vi "mainUIPumpProbe.vi"() -> ()   [LabVIEW 2017]
uses:
  globalUtilities.vi
  globalDevices.vi
panel:
  in  "axis (z)":u16(ring)=2 items=["x", "y", "z"]
  in  "length 2":i32
  in  "index 2":i32
  in  "length":i32
  in  "index":i32
  out "Waveform Graph":dbl[](graph)
  in  "saveVolume":bool
  in  "axis 1":u16(ring) items=["x", "y", "z"]
  out "frame 3":u64[][](graph)
  out "dropped frames":i32
  in  "acquisitionStart":bool
  in  "STOP":bool
  out "frame":u64[][](graph)
  in  "volume height (um)":dbl=80.0
  in  "volumes per second":dbl=0.5
  in  "GUI update divider":i32=1
  in  "frames per second":dbl=10.0
  out "folder name":string
  # "This VI sets all the acquisition parameters, starts the actual backend VI asynchronously, and displays the frames."
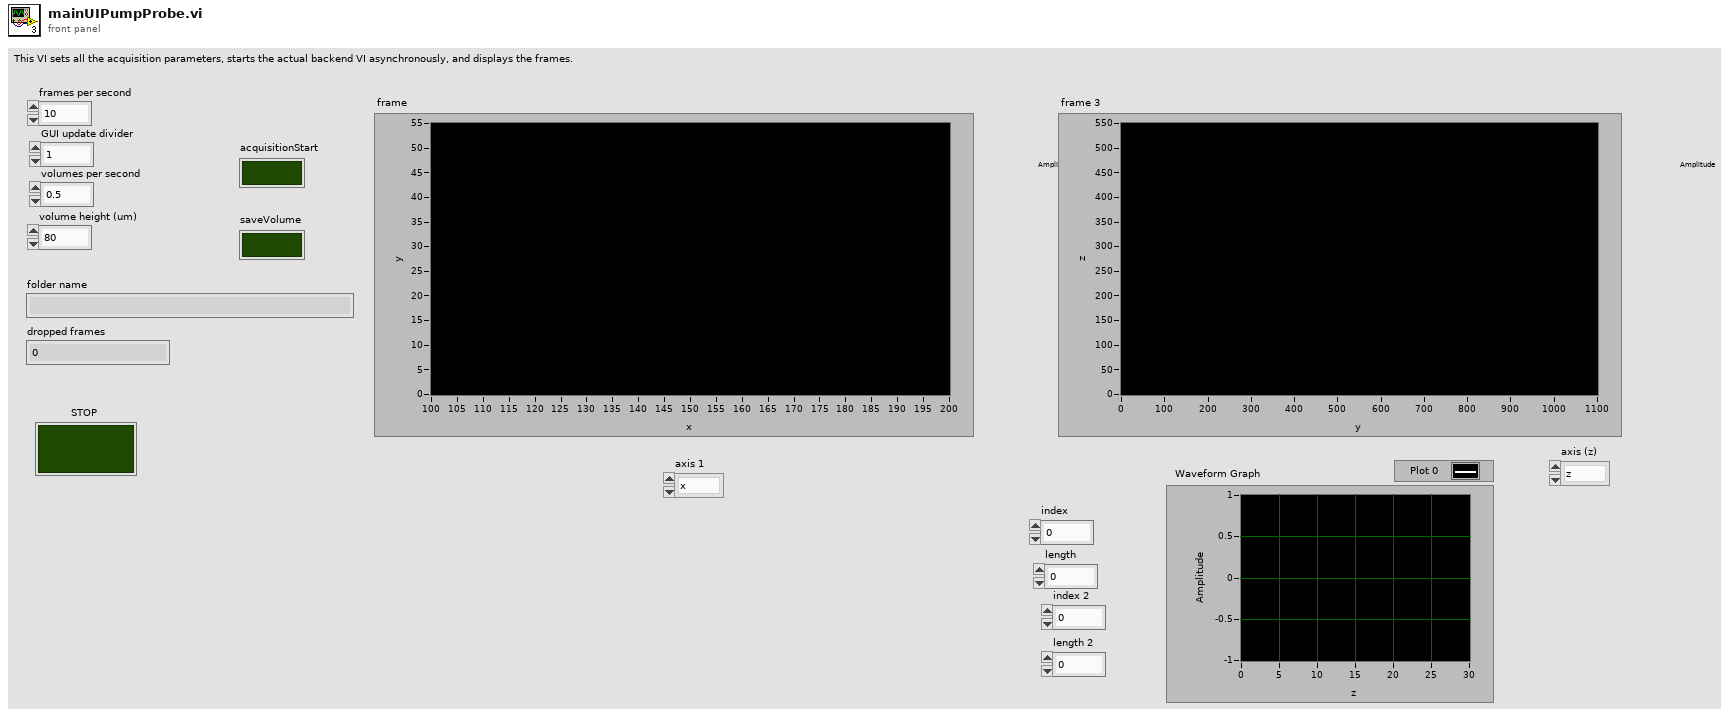
[diagram p1: front panel]
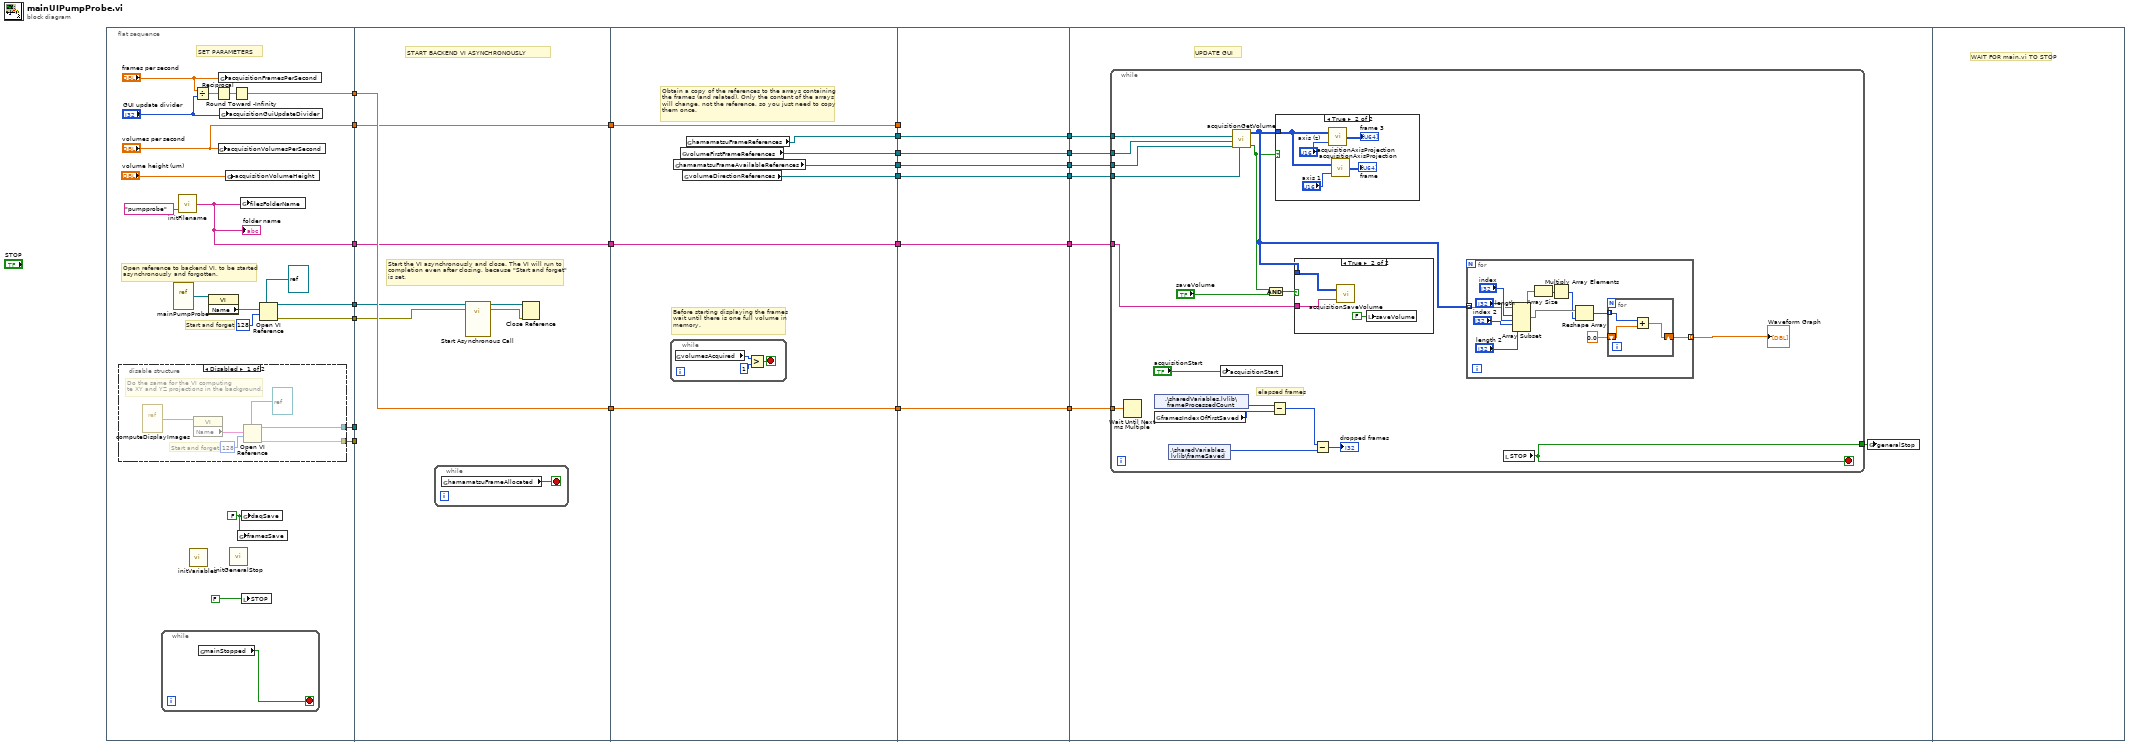
[diagram p0: block diagram]
diagram:
  n1 = flat-sequence {
    tunnel: [w37] -> w23
    tunnel: [w35] -> w22
    tunnel: [w33] -> w21
    tunnel: ["volumes per second"] -> w19
    tunnel: [w30] -> w17
    tunnel: [w29] -> w16
    tunnel: [w28] -> w15
    tunnel: w23 -> [w56]
    tunnel: [w56] -> w14
    tunnel: w22 -> [w55]
    tunnel: w21 -> [w54]
    tunnel: [w51] -> w12
    tunnel: w19 -> [w51]
    tunnel: [w50] -> w10
    tunnel: w17 -> [w50]
    tunnel: w16 -> [_]
    tunnel: w15 -> [_]
    tunnel: w14 -> [w64]
    tunnel: [w64] -> w13
    tunnel: w12 -> [w63]
    tunnel: [w63] -> w11
    tunnel: w10 -> [w62]
    tunnel: [w62] -> w9
    tunnel: [w61] -> w7
    tunnel: [w60] -> w5
    tunnel: [w59] -> w3
    tunnel: [w58] -> w1
    tunnel: w13 -> [w73]
    tunnel: [w73] -> w20
    tunnel: w11 -> [_]
    tunnel: [w72] -> w18
    tunnel: w9 -> [w72]
    tunnel: [w71] -> w8
    tunnel: w7 -> [w71]
    tunnel: [w70] -> w6
    tunnel: w5 -> [w70]
    tunnel: [w69] -> w4
    tunnel: w3 -> [w69]
    tunnel: [w68] -> w2
    tunnel: w1 -> [w68]
    tunnel: w20 -> [w80]
    tunnel: w18 -> [w78]
    tunnel: w8 -> [w77]
    tunnel: w6 -> [w76]
    tunnel: w4 -> [w75]
    tunnel: w2 -> [w74]
    frame #0 {
      w34 = FALSE ("daqSave")
      # "Start and forget"
      # "Open reference to backend VI, to be started\nasynchronously and forgotten."
      # "SET PARAMETERS"
      n2 = disable-structure shown="Disabled" {
        disable-tunnel: [w48 _] -> w29
        disable-tunnel: [w47 _] -> w28
        frame Disabled {
          # "Do the same for the VI computing\nte XY and YZ projections in the background."
          # "Start and forget"
          n3 = vi-ref "computeDisplayImages.vi"() -> (w43:refnum<vi>)
          n4 = property class="VI"(reference=w43) -> ("Name"=w46:string)  [unwired: 1 in, 2 out]
          n5 = Open VI Reference(type specifier VI Refnum (for type only)=refnum<vi> refnum, vi path=w46, options=128) -> (vi reference=w48:refnum<vi>, error out=w47:errorcluster)  [unwired: 3 in]
        }
        frame Enabled {
        }
      }
      n6 = while {
        stop <- w49 stop-if-true
        n7 = global read "globalUtilities.vi" "mainStopped"() -> (w49:bool)
      }
      n8 = vi-ref "mainPumpProbe.vi"() -> (w27:refnum<vi>)
      n9 = call "initFilename.vi"("Experiment type"="pumpprobe") -> ("folder name"=w30:string)  [unwired: 1 in]
      "folder name" <- w30
      n10 = call "initVariables.vi"() -> ()  [unwired: 12 in]
      n11 = Divide(x="frames per second", y="GUI update divider") -> (x/y=w39:dbl)
      n12 = property class="VI"(reference=w27) -> ("Name"=w26:string)  [unwired: 1 in, 2 out]
      n13 = Reciprocal(x=w39) -> (1/x=w38:dbl)
      n14 = global write "globalUtilities.vi" "acquisitionVolumesPerSecond"("volumes per second") -> ()
      n15 = global write "globalUtilities.vi" "acquisitionFramesPerSecond"("frames per second") -> ()
      n16 = global write "globalUtilities.vi" "acquisitionGuiUpdateDivider"("GUI update divider") -> ()
      n17 = global write "globalUtilities.vi" "acquisitionVolumeHeight"("volume height (um)") -> ()
      n18 = call "initGeneralStop.vi"() -> ()  [unwired: 1 in]
      n19 = Round Toward -Infinity(1:w38) -> (0:w37:dbl)
      n20 = global write "globalUtilities.vi" "framesSave"(w34) -> ()
      n21 = global write "globalUtilities.vi" "filesFolderName"(w30) -> ()
      n22 = local write "STOP"(FALSE) -> ()
      n23 = global write "globalUtilities.vi" "daqSave"(w34) -> ()
      n24 = Open VI Reference(type specifier VI Refnum (for type only)=refnum<vi> refnum, vi path=w26, options=128) -> (vi reference=w35:refnum<vi>, error out=w33:errorcluster)  [unwired: 3 in]
    }
    frame #1 {
      # "Start the VI asynchronously and close. The VI will run to\ncompletion even after closing, because \"Start and forget\"\nis set."
      # "START BACKEND VI ASYNCHRONOUSLY"
      n25 = while {
        stop <- w57 stop-if-true
        n26 = global read "globalDevices.vi" "hamamatsuFrameAllocated"() -> (w57:bool)
      }
      n27 = call-by-ref "Start Asynchronous Call"(reference=w55, error in=w54) -> (reference out=w53:refnum<vi>, error out=w52:errorcluster)  [unwired: 12 in]
      n28 = Close Reference(reference=w53, error in (no error)=w52) -> ()  [unwired: 1 out]
    }
    frame #2 {
      # "Obtain a copy of the references to the arrays containing \nthe frames (and related). Only the content of the arrays\nwill change, not the reference, so you just need to copy\nthem once."
      # "Before starting displaying the frames\nwait until there is one full volume in\nmemory."
      n29 = while {
        stop <- w66 stop-if-true
        n30 = global read "globalUtilities.vi" "volumesAcquired"() -> (w65:i32)
        n31 = Greater?(x=w65, y=1) -> (0:w66:bool)
      }
      n32 = global read "globalDevices.vi" "hamamatsuFrameAvailableReferences"() -> (w59:refnum<data-value>[])
      n33 = global read "globalUtilities.vi" "volumeFirstFrameReferences"() -> (w60:refnum<data-value>[])
      n34 = global read "globalUtilities.vi" "volumeDirectionReferences"() -> (w58:refnum<data-value>[])
      n35 = global read "globalDevices.vi" "hamamatsuFrameReferences"() -> (w61:refnum<data-value>[])
    }
    frame #3 {
    }
    frame #4 {
      # "UPDATE GUI"
      n36 = while {
        tunnel: w80 -> [w98]
        tunnel: [w91] -> w79
        tunnel: w78 -> [w90]
        tunnel: w77 -> [w87]
        tunnel: w76 -> [w86]
        tunnel: w75 -> [w85]
        tunnel: w74 -> [w84]
        stop <- w91 stop-if-true
        # "elapsed frames"
        n37 = Wait Until Next ms Multiple(millisecond multiple=w98) -> ()  [unwired: 1 out]
        n38 = shared-variable ".\\sharedVariables.lvlib\\frameProcessedCount"() -> (w96:i32)  [unwired: 1 in, 1 out]
        n39 = global read "globalUtilities.vi" "framesIndexOfFirstSaved"() -> (w95:i32)
        n40 = shared-variable ".\\sharedVariables.lvlib\\frameSaved"() -> (w93:u32)  [unwired: 1 in, 1 out]
        n41 = global write "globalUtilities.vi" "acquisitionStart"("acquisitionStart") -> ()
        n42 = call "acquisitionGetVolume.vi"("volumeDirectionReferences"=w84, "hamamatsuFrameAvailableReferences"=w85, "volumeFirstFrameReferences"=w86, "hamamatsuFrameReferences"=w87) -> ("success"=w81:bool, "volume out"=w89:u16[][][])  [unwired: 1 in, 3 out]
        n43 = And(x=w81, y="saveVolume") -> (x .and. y?=w83:bool)
        n44 = Subtract(x=w96, y=w95) -> (x-y=w94:i32)
        n45 = case shown="True" w81 {
          tunnel: w89 -> [_ w100]
          frame False {
          }
          frame True {
            n46 = call "acquisitionAxisProjection.vi"("axis (z)"="axis (z)", "z stack"=w100) -> ("projected img"=→"frame 3":u64[][])
            n47 = call "acquisitionAxisProjection.vi"("axis (z)"="axis 1", "z stack"=w100) -> ("projected img"=→"frame":u64[][])
          }
        }
        n48 = case shown="True" w83 {
          tunnel: w89 -> [_ w120]
          tunnel: w90 -> [_ w119]
          frame False {
          }
          frame True {
            n49 = call "acquisitionSaveVolume.vi"("folder"=w119, "volume"=w120) -> ()  [unwired: 1 in]
            n50 = local write "saveVolume"(FALSE ("saveVolume")) -> ()
          }
        }
        n51 = Subtract(x=w94, y=w93) -> (x-y=→"dropped frames":u32)
        n52 = for {
          tunnel: w89 -> [w110] mode=indexing
          tunnel: [w104] -> w88 mode=indexing
          n53 = Array Subset(array=w110, index (row)="index", length (row)="length", index (col)="index 2", length (col)="length 2") -> (w108:u16[][])
          n54 = Array Size(array=w108) -> (size(s)=w109:i32[])
          n55 = Multiply Array Elements(1:w109) -> (0:w107:i32)
          n56 = Reshape Array(w108, w107) -> (w106:u16[])
          n57 = for {
            tunnel: w106 -> [w117] mode=indexing
            shift-right: [w115] -> w104
            shift-left: 0.0 -> [w116]
            n58 = Add(x=w117, y=w116) -> (x+y=w115:dbl)
          }
        }
        "Waveform Graph" <- w88
        n59 = local read "STOP"() -> (w91:bool)
      }
      n60 = global write "globalUtilities.vi" "generalStop"(w79) -> ()
    }
    frame #5 {
      # "WAIT FOR main.vi TO STOP"
    }
  }
